vi "GP22_TDC_Arduinoed Measurement.vi"() -> ()   [LabVIEW 2014, in "GP22_TDC_Arduinoed.lvlib"]
uses:
  GP22_TDC_Arduinoed.lvlib
  <vilib>/Utility/file.llb/Write To Spreadsheet File (DBL).vi
  <vilib>/Analysis/NI_AALBase.lvlib
panel:
  out "Histogram":dynamicdata(graph)
  out "fractional S.D.":dbl
  out "Freq / Hz":dbl
  out "Size":i32
  out "output/s":dbl[](array[numeric]) format="%^#_6g"
  in  "Time in ms (30000)":i32=30000
  out "error out":errorcluster
  out "Self-Test Result Message":string
  in  "VISA resource name":refnum<visa-resource-name>="COM6"
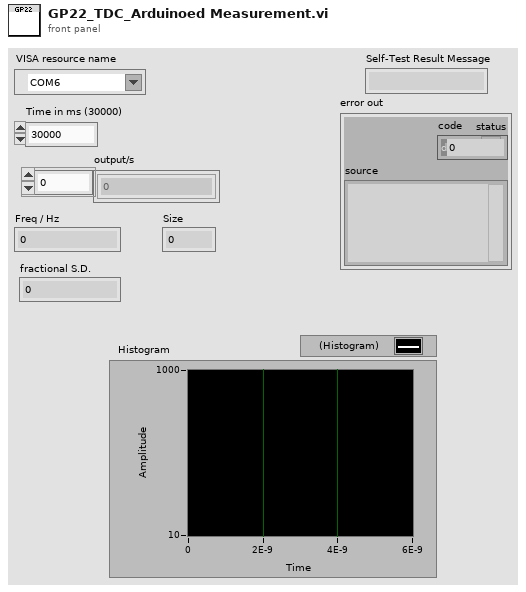
[diagram p1: front panel]
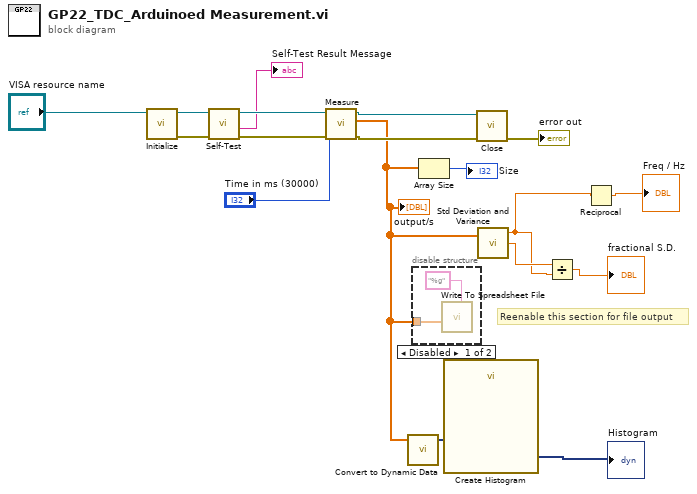
[diagram p0: block diagram]
diagram:
  # "Reenable this section for file output"
  n1 = call "Initialize.vi"("VISA resource name"="VISA resource name") -> ("error out"=w13:errorcluster, "VISA resource name out"=w16:refnum<visa-resource-name>)  [unwired: 9 in]
  n2 = call "Self-Test.vi"("error in (no error)"=w13, "VISA resource name"=w16) -> ("error out"=w14:errorcluster, "Self-Test Result Message"=→"Self-Test Result Message":string, "VISA resource name out"=w15:refnum<visa-resource-name>)  [unwired: 6 in, 1 out]
  n3 = call "Measure.vi"("Time in ms (30000)"="Time in ms (30000)", "VISA resource name"=w15) -> ("output"=w6:dbl[], "VISA resource name out"=w10:refnum<visa-resource-name>)  [unwired: 7 in, 1 out]
  "output/s" <- w6
  n4 = call "Convert to Dynamic Data"("Array"=w6) -> ("Dynamic Data Type"=w5:dynamicdata)  [unwired: 3 in]
  n5 = disable-structure shown="Disabled" {
    disable-tunnel: w6 -> [w19 _]
    frame Disabled {
      n6 = call-poly <vilib>:"Write To Spreadsheet File.vi"("format (%.3f)"="%g", "1D data"=w19) -> ()  [unwired: 6 in, 1 out]
    }
    frame Enabled {
    }
  }
  n7 = Array Size(array=w6) -> (size(s)=→"Size":i32)
  n8 = call "Create Histogram"("Signal"=w5) -> ("Histogram"=→"Histogram":dynamicdata)  [unwired: 9 in, 1 out]
  n9 = call "Close.vi"("error in (no error)"=w14, "VISA resource name"=w10) -> ("error out"=→"error out":errorcluster)  [unwired: 9 in]
  n10 = call <vilib>:"Std Deviation and Variance.vi"("X"=w6) -> ("mean"=w1:dbl, "standard deviation"=w3:dbl)  [unwired: 1 in, 1 out]
  n11 = Divide(x=w3, y=w1) -> (x/y=→"fractional S.D.":dbl)
  n12 = Reciprocal(x=w1) -> (1/x=→"Freq / Hz":dbl)
